vi "CCL_Query.vi"(0 "System no.":i32=1 min=1 max=4 step=1, 5 "error in":errorcluster) -> (14 "Command level":i32, 19 "error out":errorcluster)   [LabVIEW 2020]
doc: "Returns the current command level. \n\nC-867, C-884, Mercury_GCS: \n\nE-816: This command cannot be issued to a slave. Check controller manual to find out if CCL? is supported.\n\nC-887, F-206, M-8X0: Only for GCS syntax version = GCS 2.0 or higher (check with CSV?.vi. If CSV?.vi is not supported, syntax version is GCS 1.0)."
panel:
  # "Returns the current command level."
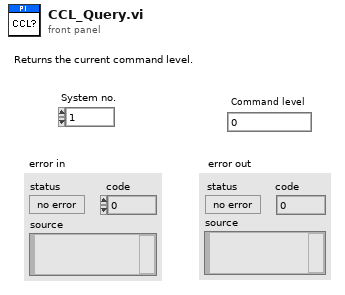
[diagram p1: front panel]
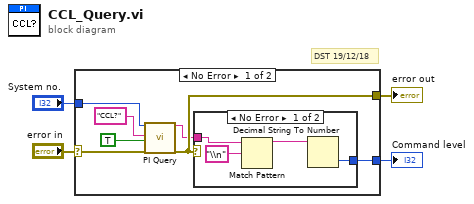
[diagram p0: block diagram]
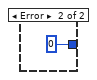
[diagram p2: hidden frame]
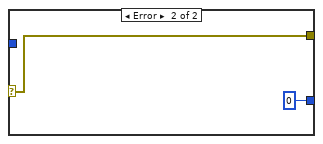
[diagram p3: hidden frame]
diagram:
  # "DST 19/12/18"
  n1 = case shown="No Error" "error in" {
    selector: "error in" -> [w7 w18]
    tunnel: [w11 0] -> w4
    tunnel: "System no." -> [w9 _]
    tunnel: [w6 w18] -> w2
    frame No Error {
      n2 = call "PI Query.vi"("System no."=w9, "String to send"="CCL?", "Attach termination char.?"=TRUE ("Attach Linefeed?"), "error in"=w7) -> ("String read"=w5:string, "error out"=w6:errorcluster)  [unwired: 3 in, 11 out]
      n3 = case shown="No Error" w6 {
        tunnel: w5 -> [w14 _]
        tunnel: [w15 0] -> w11
        frame No Error {
          n4 = Match Pattern(string=w14, regular expression="\\n") -> (before substring=w12:string)  [unwired: 4 out]
          n5 = Decimal String To Number(string=w12) -> (number=w15:i32)  [unwired: 3 out]
        }
        frame Error {
        }
      }
    }
    frame Error {
    }
  }
  "error out" <- w2
  "Command level" <- w4
